vi "myRIO__TCP_constants_byteRange_messageType_trial.vi"() -> (2 "output_Trial_byte":u8=84, 3 "output_Trial_char":string="T")   [LabVIEW 2014]
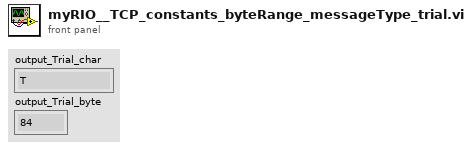
[diagram p1: front panel]
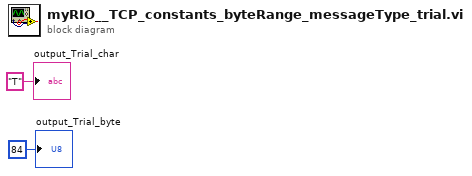
[diagram p0: block diagram]
diagram:
  "output_Trial_char" <- "T"
  "output_Trial_byte" <- u8 84
